vi "Encryption.Hex String to U8 Array.VI"(1 "Hex String":string) -> (0 "U8 Array In":u8[](array[numeric]))   [LabVIEW 2024, in "KATE_Lib.lvlib" / "Encryption.lvlib"]
uses:
  Encryption.lvlib
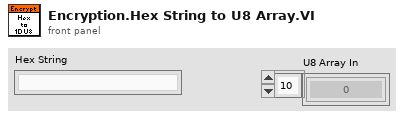
[diagram p1: front panel]
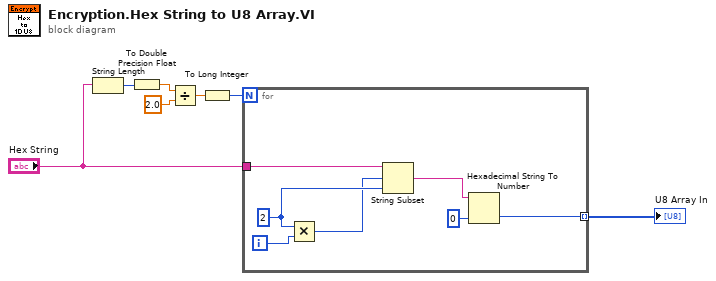
[diagram p0: block diagram]
diagram:
  n1 = String Length(string="Hex String") -> (length=w3:i32)
  n2 = To Double Precision Float(number=w3) -> (double precision float=w2:dbl)
  n3 = Divide(x=w2, y=2.0) -> (x/y=w5:dbl)
  n4 = To Long Integer(number=w5) -> (32bit integer=w4:i32)
  n5 = for {
    N: w4 -> [_]
    tunnel: "Hex String" -> [w11]
    tunnel: [w8] -> w7 mode=indexing
    i -> [w14]
    w13 = 2 ("x")
    n6 = Multiply(x=w13, y=w14) -> (x*y=w12:i32)
    n7 = String Subset(string=w11, offset (0)=w12, length (rest)=w13) -> (substring=w10:string)
    n8 = Hexadecimal String To Number(string=w10, default (0uL)=u8 0 ("default (0 U32)")) -> (number=w8:u8)  [unwired: 1 in, 1 out]
  }
  "U8 Array In" <- w7
